vi "Sync state DSP402.vi"(2 "Status":u16, 3 "DSP402 in":refnum<class "DSP402.lvclass">) -> (1 "DSP402 out":refnum<class "DSP402.lvclass">)   [LabVIEW 2024, in "canopen.lvlib" / "DSP402.lvclass"]
uses:
  DSP402.lvclass
  DSP402.lvclass/DSP402.ctl
  DriveState.ctl
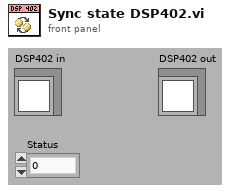
[diagram p1: front panel]
types:
  T1 = typedef "canopen.lvlib/DSP402.lvclass/DriveState.ctl" = enum16{"Start", "Not ready to switch on", "Switch on disabled", "Ready to switch on", "Switched on", "Operation enable", "Fault reaction active", "Fault", "Quick stop active"}
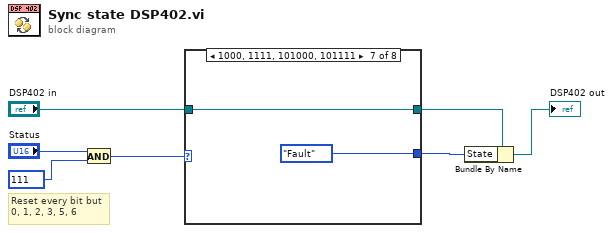
[diagram p0: block diagram]
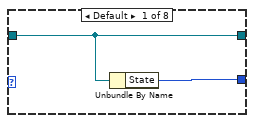
[diagram p2: hidden frame]
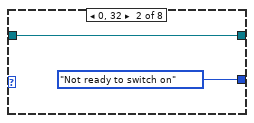
[diagram p3: hidden frame]
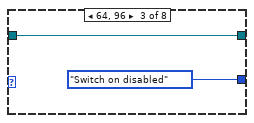
[diagram p4: hidden frame]
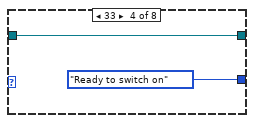
[diagram p5: hidden frame]
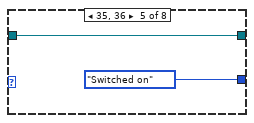
[diagram p6: hidden frame]
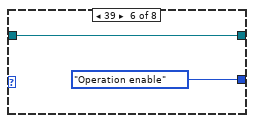
[diagram p7: hidden frame]
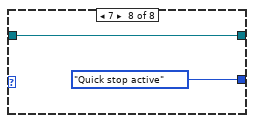
[diagram p8: hidden frame]
diagram:
  # "Reset every bit but\n0, 1, 2, 3, 5, 6"
  n1 = And(x="Status", y=u16 111 ("Index")) -> (x .and. y?=w4:u16)
  n2 = case shown="1000, 1111, 101000, 101111" w4 {
    tunnel: "DSP402 in" -> [w9 w11 w13 w15 w17 w19 w21 w23]
    tunnel: [w9 w11 w13 w15 w17 w19 w21 w23] -> w2
    tunnel: [w8 DriveState."Not ready to switch on" ("State") DriveState."Switch on disabled" ("State") DriveState."Ready to switch on" ("State") DriveState."Switched on" ("State") DriveState."Operation enable" ("State") DriveState."Fault" ("State") DriveState."Quick stop active" ("State")] -> w1
    frame Default {
      n3 = Unbundle By Name(w9) -> ("State"=w8:T1)
    }
    frame 0, 32 {
    }
    frame 64, 96 {
    }
    frame 33 {
    }
    frame 35, 36 {
    }
    frame 39 {
    }
    frame 8, 15, 40, 47 {
    }
    frame 7 {
    }
  }
  n4 = Bundle By Name(cluster=w2, "State"=w1) -> (→"DSP402 out":refnum<class "DSP402.lvclass">)
